vi "FPGA.vi"() -> ()   [LabVIEW 2018]
uses:
  <vilib>/Platform/TimedLoop/XDataNode/timing_clust.ctl
  <vilib>/Platform/TimedLoop/XDataNode/nitl_modes.ctl
  <vilib>/Platform/TimedLoop/XDataNode/wakeup.ctl
  <vilib>/rvi/Emulation/niFpgaGetClockAttributes.vi
  <vilib>/rvi/Emulation/niFpgaSctlEmulationGetInTimedLoop.vi
  <vilib>/rvi/Emulation/niFpgaEmulationReportErrorSimple.vi
  <vilib>/rvi/Emulation/niFpgaProcessEmulError.vi
  <vilib>/rvi/eio/common/nirviEmuTemplateMethod_errors.vi
  <vilib>/rvi/Emulation/niFpgaCriticalErrorInLSC.vi
  <vilib>/eio/EIONode/EIONode.xnode
  <vilib>/Platform/TimedLoop/XDataNode/XDataNode.xnode
  <vilib>/Platform/TimedLoop/XDataNode/XDNodeRunTimeDep.lvlib
  Library/jmslib.lvlib
panel:
  out "Analog":T1
  in  "Reset 1":bool
  in  "stop":bool
  in  "CH5 DC":fxp<+,32,0>
  in  "Reset 5":bool
  out "JumpBy2Error 5":i16
  out "Position 5":i32
  in  "STBY5":bool
  in  "ENA5":bool
  in  "DIR5":bool
  out "Position 1":i32
  in  "DIR4":bool
  in  "ENA4":bool
  in  "STBY4":bool
  out "Position 4":i32
  out "JumpBy2Error 4":i16
  in  "Reset4":bool
  in  "CH4 DC":fxp<+,32,0>
  in  "DIR3":bool
  in  "ENA3":bool
  in  "STBY3":bool
  out "Position 3":i32
  out "JumpBy2Error 3":i16
  in  "Reset3":bool
  in  "CH3 DC":fxp<+,32,0>
  in  "DIR2":bool
  in  "ENA2":bool
  in  "STBY2":bool
  out "Position 2":i32
  out "JumpBy2Error 2":i16
  in  "Reset 2":bool
  in  "CH2 DC":fxp<+,32,0>
  in  "CH1 DC":fxp<+,32,0>
  out "JumpBy2Error 1":i16
  in  "STBY1":bool
  in  "ENA1":bool
  in  "DIR1":bool
  # "Channel 1"
  # "Channel 2"
  # "Channel 3"
  # "Channel 4"
  # "Channel 5"
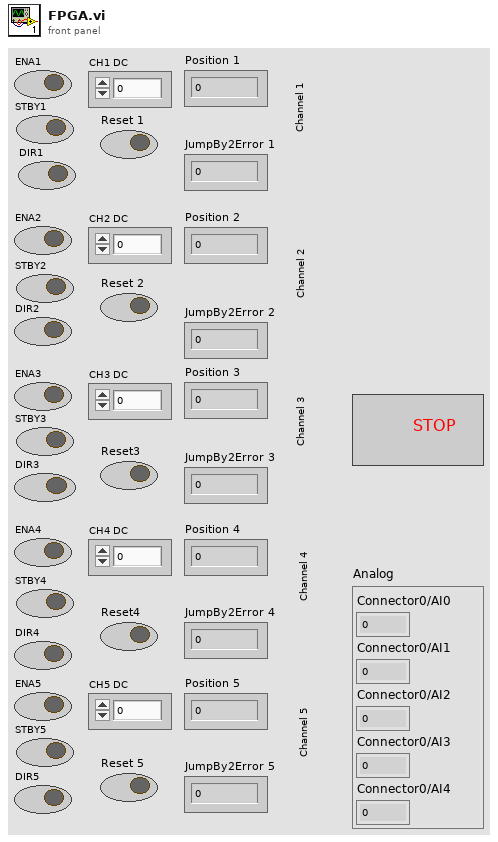
[diagram p1: front panel]
types:
  T1 = cluster{"Connector0/AI0":i16, "Connector0/AI1":i16, "Connector0/AI2":i16, "Connector0/AI3":i16, "Connector0/AI4":i16}
  T2 = typedef "XDNodeRunTimeDep.lvlib/timing_clust.ctl" = cluster{"Expected End [f-1]":u64, "Actual End [f-1]":u64, "Finished Late? [f-1]":bool, "Expected End [i-1]":u64, "Actual End [i-1]":u64, "Finished Late? [i-1]":bool, "Expected Start [i]":u64, "Actual Start [i]":u64, "Expected Start [f]":u64, "Actual Start [f]":u64, "Source Name":string, "Structure Name":string, "Period":i64, "Deadline":i64, "Offset":i64, "Start":i64, "Priority":i32, "Timeout":i32, "Mode":T3, "Wakeup Reason":T4, "Error":errorcluster, "Source Type":string, "Secondary Source Type":string, "Global End Time":u64, "Global Start Time":u64, "Frame Duration":u64, "Iteration Duration":u64, "Assigned CPU":i32, "I/O Scan Engine Mode":u32}
  T3 = typedef "XDNodeRunTimeDep.lvlib/nitl_modes.ctl" = enum32{"No Change", "Process missed periods, maintain original phase", "Discard missed periods, maintain original phase", "Process missed periods, ignore original phase", "Discard missed periods, ignore original phase"}
  T4 = typedef "XDNodeRunTimeDep.lvlib/wakeup.ctl" = enum32{"Normal", "Aborted", "Asynchronous wakeup", "Timing source error", "Timed loop error", "Timeout"}
  T5 = cluster{"PWM In":refnum<k21>, "Direction":refnum<k21>, "Inhibit":refnum<k21>, "Encoder C":refnum<k21>, "Encoder B":refnum<k21>, "Encoder A":refnum<k21>, "Fault":refnum<k21>}
  T6 = cluster{"I/O Item":i16, "I/O Item":i16, "I/O Item":i16, "Connector0/AI3":i16, "Connector0/AI4":i16}
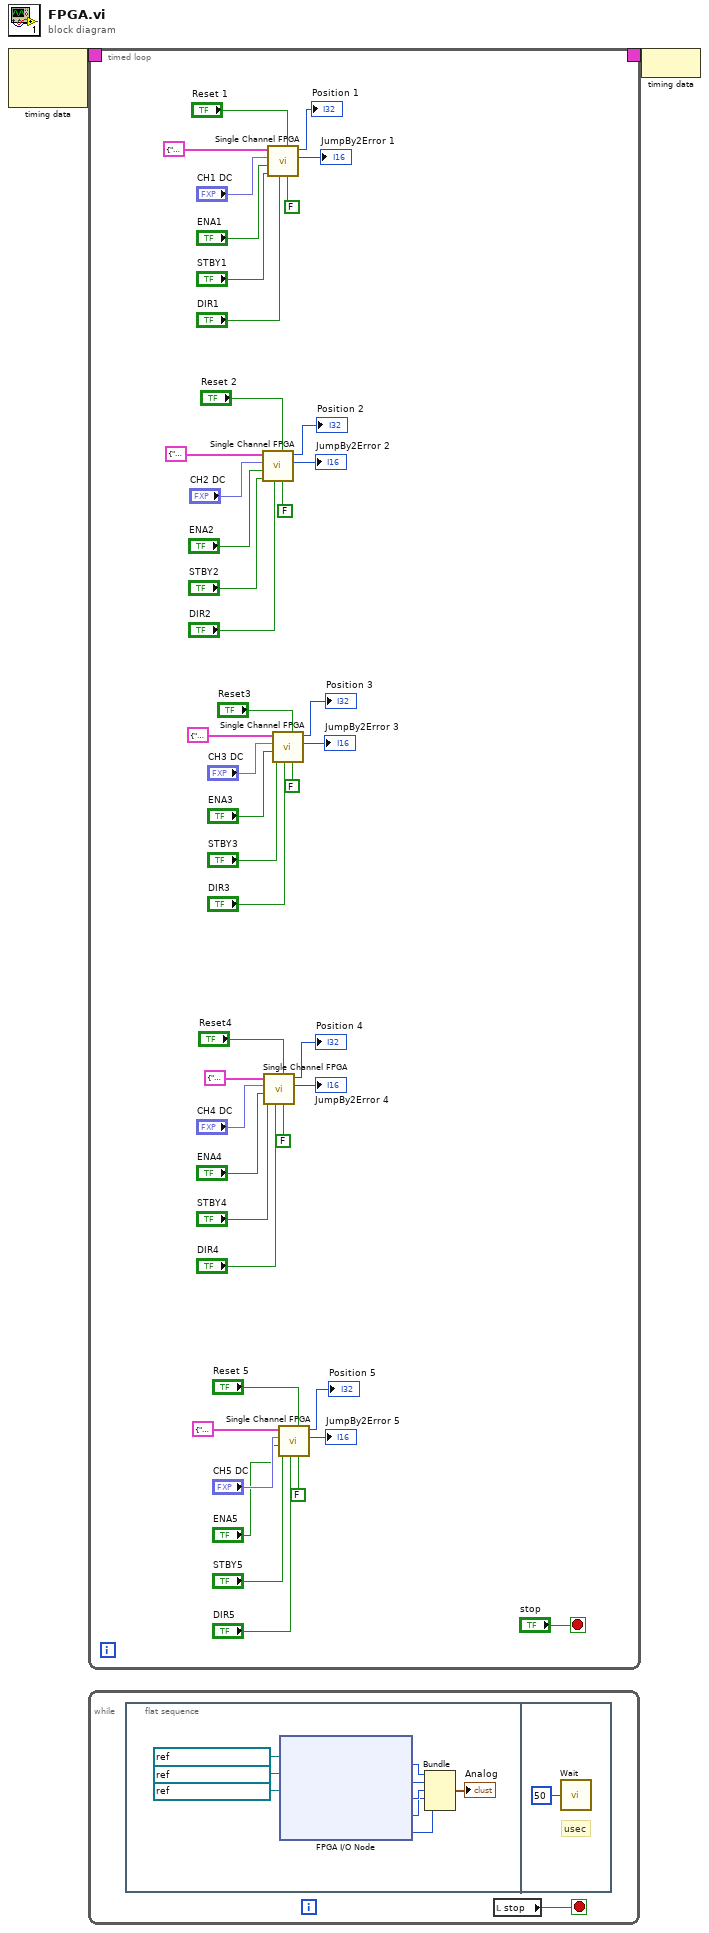
[diagram p0: block diagram]
diagram:
  n1 = node-c288() -> (w2:T2)  [unwired: 2 in]
  n2 = timed-loop {
    timing: w2 -> [_]
    timing-out: [_] -> w1
    stop <- "stop" stop-if-true
    n3 = call "Single Channel FPGA.vi"("Reset by Enc C"=FALSE, "Reset by hand"="Reset 2", "DIR"="DIR2", "STBY"="STBY2", "ENA"="ENA2", "Duty"="CH2 DC", "IO Channels"=T5 {"PWM In"="Connector1/DIO1", "Direction"="Connector1/DIO2", "Inhibit"="Connector1/DIO3", "Encoder C"="Connector1/DIO4", "Encoder B"="Connector1/DIO5", "Encoder A"="Connector1/DIO6", "Fault"="Connector1/DIO0"}) -> ("JumpBy2Error"=→"JumpBy2Error 2":i16, "Position"=→"Position 2":i32)  [unwired: 3 in]
    n4 = call "Single Channel FPGA.vi"("Reset by Enc C"=FALSE, "Reset by hand"="Reset4", "DIR"="DIR4", "STBY"="STBY4", "ENA"="ENA4", "Duty"="CH4 DC", "IO Channels"=T5 {"PWM In"="Connector1/DIO14", "Direction"="Connector1/DIO15", "Inhibit"="Connector1/DIO16", "Encoder C"="Connector1/DIO17", "Encoder B"="Connector1/DIO18", "Encoder A"="Connector1/DIO19", "Fault"="Connector1/DIO26"}) -> ("JumpBy2Error"=→"JumpBy2Error 4":i16, "Position"=→"Position 4":i32)  [unwired: 3 in]
    n5 = call "Single Channel FPGA.vi"("Reset by Enc C"=FALSE, "Reset by hand"="Reset 1", "DIR"="DIR1", "STBY"="STBY1", "ENA"="ENA1", "Duty"="CH1 DC", "IO Channels"=T5 {"PWM In"="Connector1/DIO7", "Direction"="Connector1/DIO8", "Inhibit"="Connector1/DIO9", "Encoder C"="Connector1/DIO10", "Encoder B"="Connector1/DIO11", "Encoder A"="Connector1/DIO12", "Fault"="Connector1/DIO13"}) -> ("JumpBy2Error"=→"JumpBy2Error 1":i16, "Position"=→"Position 1":i32)  [unwired: 3 in]
    n6 = call "Single Channel FPGA.vi"("Reset by Enc C"=FALSE, "Reset by hand"="Reset3", "DIR"="DIR3", "STBY"="STBY3", "ENA"="ENA3", "Duty"="CH3 DC", "IO Channels"=T5 {"PWM In"="Connector1/DIO20", "Direction"="Connector1/DIO21", "Inhibit"="Connector1/DIO22", "Encoder C"="Connector1/DIO23", "Encoder B"="Connector1/DIO24", "Encoder A"="Connector1/DIO25", "Fault"="Connector1/DIO27"}) -> ("JumpBy2Error"=→"JumpBy2Error 3":i16, "Position"=→"Position 3":i32)  [unwired: 3 in]
    n7 = call "Single Channel FPGA.vi"("Reset by Enc C"=FALSE, "Reset by hand"="Reset 5", "DIR"="DIR5", "STBY"="STBY5", "ENA"="ENA5", "Duty"="CH5 DC", "IO Channels"=T5 {"PWM In"="Connector1/DIO29", "Direction"="Connector1/DIO31", "Inhibit"="Connector1/DIO33", "Encoder C"="Connector1/DIO35", "Encoder B"="Connector1/DIO37", "Encoder A"="Connector1/DIO39", "Fault"="Connector1/DIO38"}) -> ("JumpBy2Error"=→"JumpBy2Error 5":i16, "Position"=→"Position 5":i32)  [unwired: 3 in]
  }
  n8 = while {
    stop <- w51 stop-if-true
    n9 = flat-sequence {
      frame #0 {
        n10 = xnode "FPGA I/O Node"("FPGA I/O In"=refnum<k21> "Connector0/AI0", "FPGA I/O In"=refnum<k21> "Connector0/AI1", "FPGA I/O In"=refnum<k21> "Connector0/AI2") -> ("I/O Item"=w60:i16, "I/O Item"=w59:i16, "I/O Item"=w58:i16, "Connector0/AI3"=w57:i16, "Connector0/AI4"=w56:i16)  [unwired: 2 in, 5 out]
        n11 = Bundle("I/O Item"=w60, "I/O Item"=w59, "I/O Item"=w58, "Connector0/AI3"=w57, "Connector0/AI4"=w56) -> (→"Analog":T6)  [unwired: 1 in]
      }
      frame #1 {
        # "usec"
        n12 = call "Wait"("Count(uSec)"=u32 50 ("Count(mSec)")) -> ()  [unwired: 1 out]
      }
    }
    n13 = local read "stop"() -> (w51:bool)
  }
  n14 = node-c288(w1) -> ()
